vi "Read Encoder.vi"(11 "ValveModbus in":refnum<class "NeedleValve.lvclass">) -> (2 "Encoder":i32, 3 "ValveModbus out":refnum<class "NeedleValve.lvclass">)   [LabVIEW 2019, in "NeedleValve.lvclass"]
uses:
  NeedleValve.lvclass
  NeedleValve.lvclass/NeedleValve.ctl
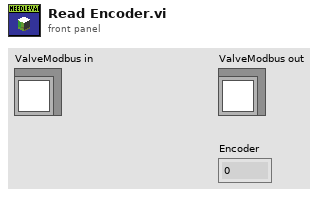
[diagram p1: front panel]
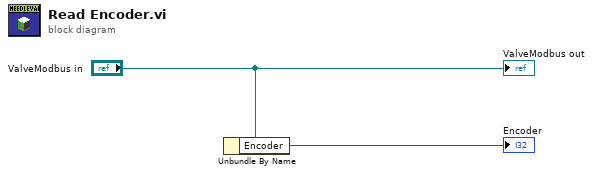
[diagram p0: block diagram]
diagram:
  n1 = Unbundle By Name("ValveModbus in") -> ("Encoder"=→"Encoder":i32)
  "ValveModbus out" <- "ValveModbus in"
